vi "pan fourtrack.vi"(7 "Track Controls":T1 {"Track 3"."Volume Settings"."Volume" scale=0.01..10.0; "Track 3"."Volume Settings"."Pan" scale=0.0..1.0; "Track 3"."Effects Settings"."Delay 2" scale=0.0..10.0; "Track 3"."Effects Settings"."Delay" scale=0.0..1.0; "Track 2"."Volume Settings"."Volume" scale=0.01..10.0; "Track 2"."Volume Settings"."Pan" scale=0.0..1.0; "Track 2"."Effects Settings"."Delay 2" scale=0.0..10.0; "Track 2"."Effects Settings"."Delay" scale=0.0..1.0; "Track 1"."Volume Settings"."Volume" scale=0.01..10.0; "Track 1"."Volume Settings"."Pan" scale=0.0..1.0; "Track 1"."Effects Settings"."Delay 2" scale=0.0..10.0; "Track 1"."Effects Settings"."Delay" scale=0.0..1.0; "Track 0"."Volume Settings"."Volume" scale=0.01..10.0; "Track 0"."Volume Settings"."Pan" scale=0.0..1.0; "Track 0"."Effects Settings"."Delay 2" scale=0.0..10.0; "Track 0"."Effects Settings"."Delay" scale=0.0..1.0}, 11 "4-Track Audio in":T5) -> (3 "4-Track Audio out":T5)   [LabVIEW 2014]
uses:
  Controls/4 Track Audio.ctl
  Controls/Audio In.ctl
  Controls/Track Controls.ctl
  Controls/Track Settings.ctl
  Controls/Track Effects Settings.ctl
  Controls/Track Volume Settings.ctl
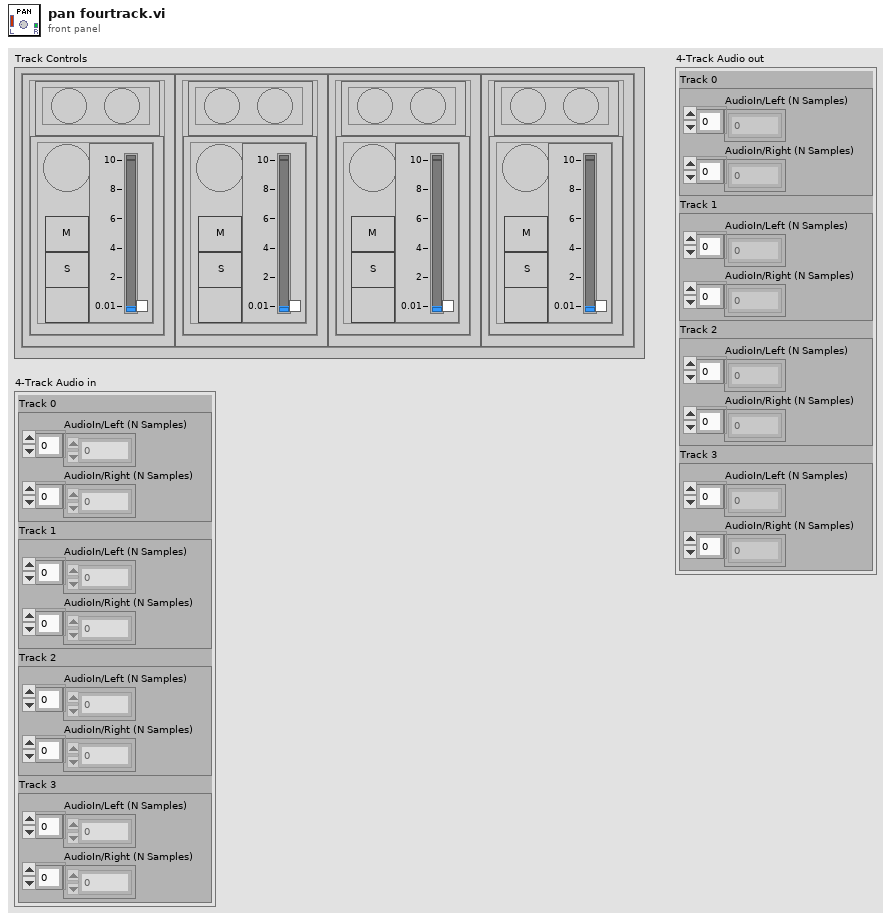
[diagram p1: front panel]
types:
  T1 = typedef "Track Controls.ctl" = cluster{"Track 0":T2, "Track 1":T2, "Track 2":T2, "Track 3":T2}
  T2 = typedef "Track Settings.ctl" = cluster{"Effects Settings":T3, "Volume Settings":T4}
  T3 = typedef "Track Effects Settings.ctl" = cluster{"Delay":dbl, "Delay 2":dbl}
  T4 = typedef "Track Volume Settings.ctl" = cluster{"Mute":bool, "Solo":bool, "Record":bool, "Pan":dbl, "Volume":dbl}
  T5 = typedef "4 Track Audio.ctl" = cluster{"Track 0":T6, "Track 1":T6, "Track 2":T6, "Track 3":T6}
  T6 = typedef "Audio In.ctl" = cluster{"AudioIn/Left (N Samples)":i16[], "AudioIn/Right (N Samples)":i16[]}
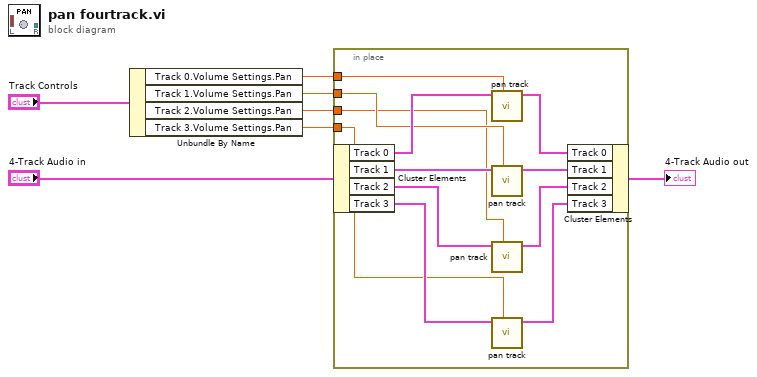
[diagram p0: block diagram]
diagram:
  n1 = Unbundle By Name("Track Controls") -> ("Track 0.Volume Settings.Pan"=w4:dbl, "Track 1.Volume Settings.Pan"=w3:dbl, "Track 2.Volume Settings.Pan"=w2:dbl, "Track 3.Volume Settings.Pan"=w1:dbl)
  n2 = in-place {
    in-place-border: w4 -> [w18]
    in-place-border: w3 -> [w17]
    in-place-border: w2 -> [w9]
    in-place-border: w1 -> [w8]
    n3 = in-place-cluster #1("4-Track Audio in") -> ("Track 0"=w19:T6, "Track 1"=w16:T6, "Track 2"=w13:T6, "Track 3"=w11:T6)
    n4 = call "pan track.vi"("Knob"=w18, "Track In"=w19) -> ("Track Out"=w15:T6)  [unwired: 9 in]
    n5 = call "pan track.vi"("Knob"=w17, "Track In"=w16) -> ("Track Out"=w14:T6)  [unwired: 9 in]
    n6 = call "pan track.vi"("Knob"=w9, "Track In"=w13) -> ("Track Out"=w12:T6)  [unwired: 9 in]
    n7 = call "pan track.vi"("Knob"=w8, "Track In"=w11) -> ("Track Out"=w10:T6)  [unwired: 9 in]
    n8 = in-place-cluster #1("Track 0"=w15, "Track 1"=w14, "Track 2"=w12, "Track 3"=w10) -> (→"4-Track Audio out":T5)
  }
